vi "System Clock to External Clock.vi"(8 "error in (no error)":errorcluster, 9 "ClockID":u8, 10 "System Time":i64, 11 "CIFCorePlugin in":refnum<class "CIFCorePlugin.lvclass">) -> (0 "error out":errorcluster, 1 "Last Reset Time":i64, 2 "External Time":i64, 3 "CIFCorePlugin out":refnum<class "CIFCorePlugin.lvclass">)   [LabVIEW 2021, in "CIFCorePlugin.lvclass"]
uses:
  CIFCorePlugin.lvclass
  CIFCorePlugin.lvclass/CIFCorePlugin.ctl
  <vilib>/CIF Foundation/CIF Utilities/Time/SubVIs/Add Error.vi
  <vilib>/CIF Foundation/CIF Utilities/Errors/Append Error Location.vi
  <vilib>/CIF Foundation/CIF Utilities/Time/Time_CIF_U.lvlib
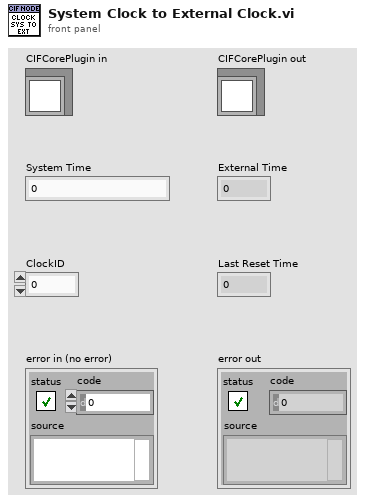
[diagram p1: front panel]
types:
  T1 = typedef "Time_CIF_U.lvlib/Clock Conversion Map.ctl" = map{u8, cluster{"Last Reset":i64, "Offset Pair":T2, "Slope":dbl, "1/Slope":dbl}}
  T2 = typedef "Time_CIF_U.lvlib/Timestamp Pair.ctl" = cluster{"System Time":i64, "External Time":i64}
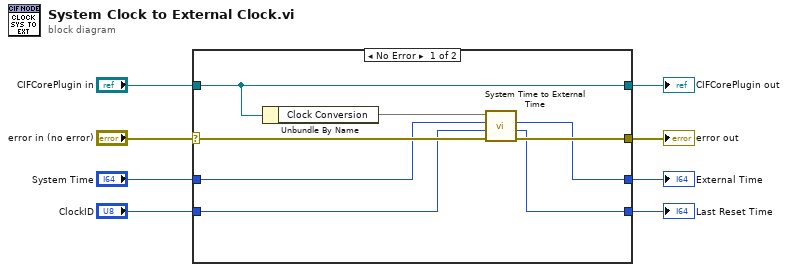
[diagram p0: block diagram]
diagram:
  n1 = case shown="No Error" "error in (no error)" {
    selector: "error in (no error)" -> [w16 w19]
    tunnel: [w15 w19] -> w7
    tunnel: [w9 w18] -> w5
    tunnel: "CIFCorePlugin in" -> [w9 w18]
    tunnel: [w14 w17] -> w4
    tunnel: "System Time" -> [w13 w17]
    tunnel: "ClockID" -> [w12 _]
    tunnel: [w11 _] -> w1
    frame No Error {
      n2 = Unbundle By Name(w9) -> ("Clock Conversion"=w10:T1)
      n3 = call <vilib>:"System Time to External Time.vi"("error in (no error)"=w16, "ClockID"=w12, "System Time"=w13, "Clock Convert Map in"=w10) -> ("error out"=w15:errorcluster, "Last Reset Time"=w11:i64, "External Time"=w14:i64)  [unwired: 4 in, 1 out]
    }
    frame Error {
    }
  }
  "error out" <- w7
  "CIFCorePlugin out" <- w5
  "External Time" <- w4
  "Last Reset Time" <- w1
